vi "_XNET Close All.vi"(8 "all classes":u32[](array[numeric]), 9 "all names":string[](array[string]), 10 "status code in":i32) -> (3 "status code out":i32)   [LabVIEW 2018]
uses:
  nixlvapi.dll
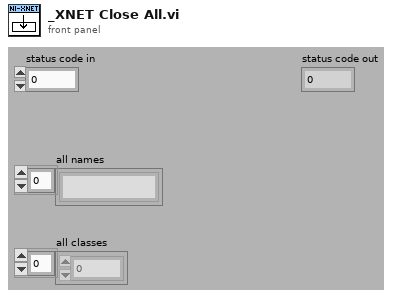
[diagram p1: front panel]
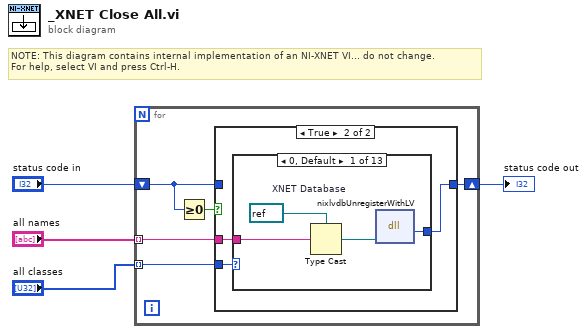
[diagram p0: block diagram]
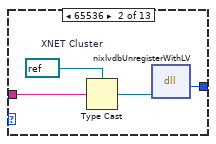
[diagram p3: hidden frame]
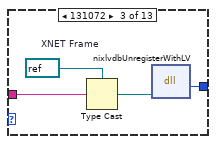
[diagram p4: hidden frame]
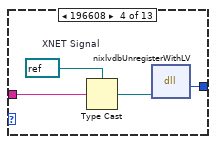
[diagram p5: hidden frame]
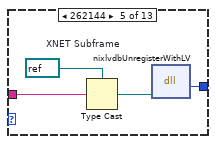
[diagram p6: hidden frame]
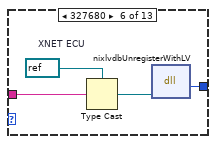
[diagram p7: hidden frame]
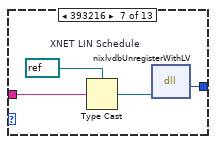
[diagram p8: hidden frame]
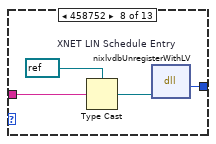
[diagram p9: hidden frame]
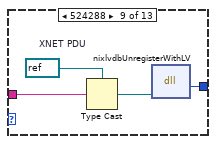
[diagram p10: hidden frame]
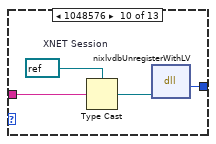
[diagram p11: hidden frame]
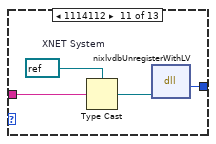
[diagram p12: hidden frame]
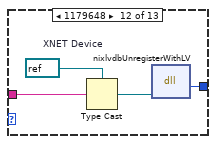
[diagram p13: hidden frame]
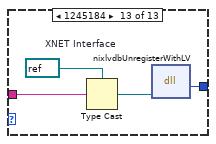
[diagram p14: hidden frame]
diagram:
  # "NOTE: This diagram contains internal implementation of an NI-XNET VI... do not change.\nFor help, select VI and press Ctrl-H."
  n1 = for {
    tunnel: "all names" -> [w7] mode=indexing
    tunnel: "all classes" -> [w8] mode=indexing
    shift-right: [w5] -> w3
    shift-left: "status code in" -> [w6]
    n2 = Greater Or Equal To 0?(x=w6) -> (x >= 0?=w9:bool)
    n3 = case shown="True" w9 {
      tunnel: w8 -> [_ w13]
      tunnel: w7 -> [_ w12]
      tunnel: w6 -> [w10 _]
      tunnel: [w10 w11] -> w5
      frame False {
      }
      frame True {
        n4 = case shown="0, Default" w13 {
          tunnel: w12 -> [w15 w19 w23 w27 w31 w35 w39 w43 w47 w51 w55 w59 w63]
          tunnel: [w17 w21 w25 w29 w33 w37 w41 w45 w49 w53 w57 w61 w65] -> w11
          frame 0, Default {
            w14 = refnum<k21> refnum  # XNET Database
            n5 = Type Cast(type=w14, x=w15) -> (*(type *) &x=w16:refnum<k21>)
            n6 = dll-call lib="nixlvapi.*" fn="nixlvdbUnregisterWithLV" ("nilvxaiu.dll:lvxenDatabaseDeleteObject")("refObjPtr"=w16) -> ("return type"=w17:i32)  [unwired: 4 in, 2 out]
          }
          frame 65536 {
            w18 = refnum<k21> refnum  # XNET Cluster
            n7 = Type Cast(type=w18, x=w19) -> (*(type *) &x=w20:refnum<k21>)
            n8 = dll-call lib="nixlvapi.*" fn="nixlvdbUnregisterWithLV" ("nilvxaiu.dll:lvxenDatabaseDeleteObject")("refObjPtr"=w20) -> ("return type"=w21:i32)  [unwired: 4 in, 2 out]
          }
          frame 131072 {
            w22 = refnum<k21> refnum  # XNET Frame
            n9 = Type Cast(type=w22, x=w23) -> (*(type *) &x=w24:refnum<k21>)
            n10 = dll-call lib="nixlvapi.*" fn="nixlvdbUnregisterWithLV" ("nilvxaiu.dll:lvxenDatabaseDeleteObject")("refObjPtr"=w24) -> ("return type"=w25:i32)  [unwired: 4 in, 2 out]
          }
          frame 196608 {
            w26 = refnum<k21> refnum  # XNET Signal
            n11 = Type Cast(type=w26, x=w27) -> (*(type *) &x=w28:refnum<k21>)
            n12 = dll-call lib="nixlvapi.*" fn="nixlvdbUnregisterWithLV" ("nilvxaiu.dll:lvxenDatabaseDeleteObject")("refObjPtr"=w28) -> ("return type"=w29:i32)  [unwired: 4 in, 2 out]
          }
          frame 262144 {
            w30 = refnum<k21> refnum  # XNET Subframe
            n13 = Type Cast(type=w30, x=w31) -> (*(type *) &x=w32:refnum<k21>)
            n14 = dll-call lib="nixlvapi.*" fn="nixlvdbUnregisterWithLV" ("nilvxaiu.dll:lvxenDatabaseDeleteObject")("refObjPtr"=w32) -> ("return type"=w33:i32)  [unwired: 4 in, 2 out]
          }
          frame 327680 {
            w34 = refnum<k21> refnum  # XNET ECU
            n15 = Type Cast(type=w34, x=w35) -> (*(type *) &x=w36:refnum<k21>)
            n16 = dll-call lib="nixlvapi.*" fn="nixlvdbUnregisterWithLV" ("nilvxaiu.dll:lvxenDatabaseDeleteObject")("refObjPtr"=w36) -> ("return type"=w37:i32)  [unwired: 4 in, 2 out]
          }
          frame 393216 {
            w38 = refnum<k21> refnum  # XNET LIN Schedule
            n17 = Type Cast(type=w38, x=w39) -> (*(type *) &x=w40:refnum<k21>)
            n18 = dll-call lib="nixlvapi.*" fn="nixlvdbUnregisterWithLV" ("nilvxaiu.dll:lvxenDatabaseDeleteObject")("refObjPtr"=w40) -> ("return type"=w41:i32)  [unwired: 4 in, 2 out]
          }
          frame 458752 {
            w42 = refnum<k21> refnum  # XNET LIN Schedule Entry
            n19 = Type Cast(type=w42, x=w43) -> (*(type *) &x=w44:refnum<k21>)
            n20 = dll-call lib="nixlvapi.*" fn="nixlvdbUnregisterWithLV" ("nilvxaiu.dll:lvxenDatabaseDeleteObject")("refObjPtr"=w44) -> ("return type"=w45:i32)  [unwired: 4 in, 2 out]
          }
          frame 524288 {
            w46 = refnum<k21> refnum  # XNET PDU
            n21 = Type Cast(type=w46, x=w47) -> (*(type *) &x=w48:refnum<k21>)
            n22 = dll-call lib="nixlvapi.*" fn="nixlvdbUnregisterWithLV" ("nilvxaiu.dll:lvxenDatabaseDeleteObject")("refObjPtr"=w48) -> ("return type"=w49:i32)  [unwired: 4 in, 2 out]
          }
          frame 1048576 {
            w50 = refnum<k21> refnum  # XNET Session
            n23 = Type Cast(type=w50, x=w51) -> (*(type *) &x=w52:refnum<k21>)
            n24 = dll-call lib="nixlvapi.*" fn="nixlvdbUnregisterWithLV" ("nilvxaiu.dll:lvxenDatabaseDeleteObject")("refObjPtr"=w52) -> ("return type"=w53:i32)  [unwired: 4 in, 2 out]
          }
          frame 1114112 {
            w54 = refnum<k21> refnum  # XNET System
            n25 = Type Cast(type=w54, x=w55) -> (*(type *) &x=w56:refnum<k21>)
            n26 = dll-call lib="nixlvapi.*" fn="nixlvdbUnregisterWithLV" ("nilvxaiu.dll:lvxenDatabaseDeleteObject")("refObjPtr"=w56) -> ("return type"=w57:i32)  [unwired: 4 in, 2 out]
          }
          frame 1179648 {
            w58 = refnum<k21> refnum  # XNET Device
            n27 = Type Cast(type=w58, x=w59) -> (*(type *) &x=w60:refnum<k21>)
            n28 = dll-call lib="nixlvapi.*" fn="nixlvdbUnregisterWithLV" ("nilvxaiu.dll:lvxenDatabaseDeleteObject")("refObjPtr"=w60) -> ("return type"=w61:i32)  [unwired: 4 in, 2 out]
          }
          frame 1245184 {
            w62 = refnum<k21> refnum  # XNET Interface
            n29 = Type Cast(type=w62, x=w63) -> (*(type *) &x=w64:refnum<k21>)
            n30 = dll-call lib="nixlvapi.*" fn="nixlvdbUnregisterWithLV" ("nilvxaiu.dll:lvxenDatabaseDeleteObject")("refObjPtr"=w64) -> ("return type"=w65:i32)  [unwired: 4 in, 2 out]
          }
        }
      }
    }
  }
  "status code out" <- w3
